vi "svc_Window Parameters.vi"(9 "standard deviation":dbl=nan format="%.2f", 10 "window size":i32, 11 "window":T1 items=["Rectangle"=0, "Hanning"=1, "Hamming"=2, "Blackman-Harris"=3, "Exact Blackman"=4, "Blackman"=5, "Flat Top"=6, "4 Term B-Harris "=7, "7 Term B-Harris"=8, "Low Sidelobe"=9, "Blackman Nuttall"=11, "Triangle"=30, "Bartlett-Hanning"=31, "Bohman"=32, "Parzen"=33, "Welch"=34, "Kaiser"=60, "Dolph-Chebyshev"=61, "Gaussian"=62]) -> (0 "maximum BW":dbl format="%.4f", 1 "6dB BW":dbl format="%.4f", 2 "Coherent Gain":dbl format="%.4f", 3 "ENBW":dbl format="%.4f")   [LabVIEW 2017]
uses:
  <vilib>/Analysis/4window.llb/windowTd.ctl
  <vilib>/Analysis/4window.llb/Window Properties by Name.vi
  <vilib>/Analysis/NI_AALPro.lvlib
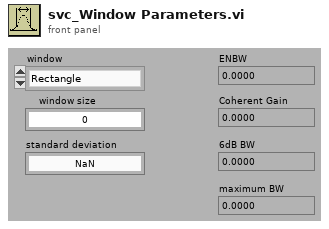
[diagram p1: front panel]
types:
  T1 = typedef "NI_AALPro.lvlib/windowTd.ctl" = u32
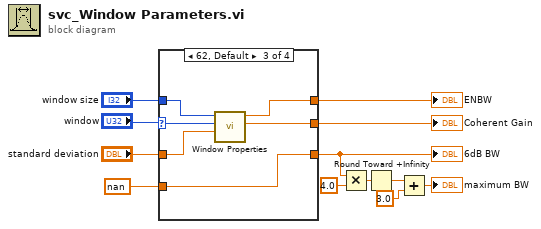
[diagram p0: block diagram]
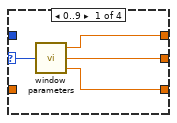
[diagram p2: hidden frame]
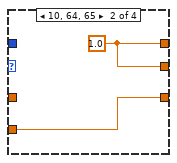
[diagram p3: hidden frame]
diagram:
  n1 = case shown="62, Default" "window" {
    selector: "window" -> [w16 _ w22 _]
    tunnel: [w14 w18 w19 w25] -> w11
    tunnel: [w15 w18 w20 w25] -> w12
    tunnel: [w13 w17 w24 w25] -> w6
    tunnel: "standard deviation" -> [_ _ w21 _]
    tunnel: "window size" -> [_ _ w23 _]
    tunnel: nan ("6dB BW") -> [_ w17 w24 w25]
    frame 0..9 {
      n2 = call <vilib>:"window parameters.vi"("window"=w16) -> ("ENBW"=w15:dbl, "Coherent Gain"=w14:dbl, "6dB BW"=w13:dbl)
    }
    frame 10, 64, 65 {
      w18 = 1.0
    }
    frame 62, Default {
      n3 = call-poly <vilib>:"Window Properties.vi"("window parameter"=w21, "window"=w22, "size"=w23) -> ("coherent gain"=w19:dbl, "eq noise BW"=w20:dbl)  [unwired: 6 in, 1 out]
    }
    frame 99 {
    }
  }
  "ENBW" <- w12
  "Coherent Gain" <- w11
  "6dB BW" <- w6
  n4 = Multiply(x=w6, y=4.0) -> (x*y=w4:dbl)
  n5 = Round Toward +Infinity(x=w4) -> (ceil(x): smallest int >= x=w3:dbl)
  n6 = Add(x=w3, y=3.0) -> (x+y=→"maximum BW":dbl)
